vi "Get AccessType.vi"(8 "error in":errorcluster, 11 "Object Type in":refnum<class "Object Type Base.lvclass">) -> (0 "error out":errorcluster, 1 "Defined?":bool, 2 "AccessType":T1=enum."const", 3 "Object Type out":refnum<class "Object Type Base.lvclass">)   [LabVIEW 2019, in "Electronic Datasheet.lvlib" / "Object Type Base.lvclass"]
uses:
  Object Type Base.lvclass
  Object Type Base.lvclass/Object Type Base.ctl
  Access Type.ctl
  Electronic Datasheet.lvlib
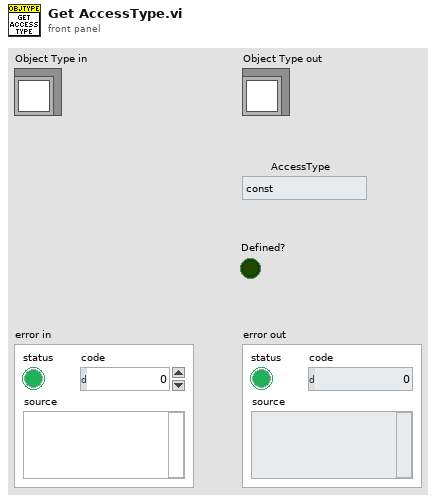
[diagram p1: front panel]
types:
  T1 = typedef "Electronic Datasheet.lvlib/Access Type.ctl" = enum16{"ro", "wo", "rw", "rwr", "rww", "const"}
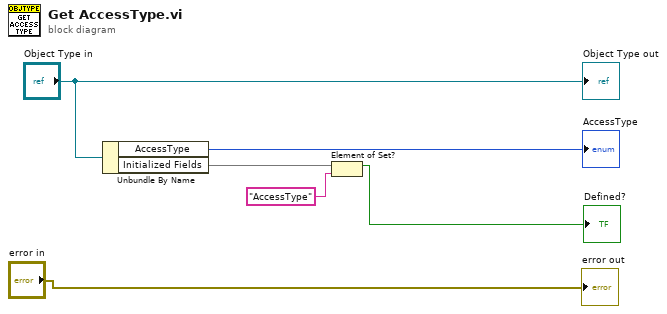
[diagram p0: block diagram]
diagram:
  n1 = Unbundle By Name("Object Type in") -> ("AccessType"=→"AccessType":T1, "Initialized Fields"=w4:set{string})
  n2 = Element of Set?(10:"AccessType" ("element"), 11:w4) -> (3:→"Defined?":bool)
  "Object Type out" <- "Object Type in"
  "error out" <- "error in"
